vi "toSplitStringArray.vi"(8 "error in (no error)":errorcluster, 9 "editing?":bool=TRUE, 10 "splitIndex":i32, 11 "ScriptEventList in":refnum<class "ScriptEventList.lvclass">) -> (0 "error out":errorcluster, 1 "AfterIndex":string[][](array[string]), 2 "BeforeIndex":string[][](array[string]), 3 "ScriptEventList out":refnum<class "ScriptEventList.lvclass">, 4 "indexedScriptEvent":refnum<class "ScriptEvent.lvclass">)   [LabVIEW 2009, in "Tools.lvlib" / "Scripting.lvlib" / "ScriptEventList.lvclass"]
uses:
  ScriptEventList.lvclass
  ScriptEvent.lvclass
  ScriptEventList.lvclass/ScriptEventList.ctl
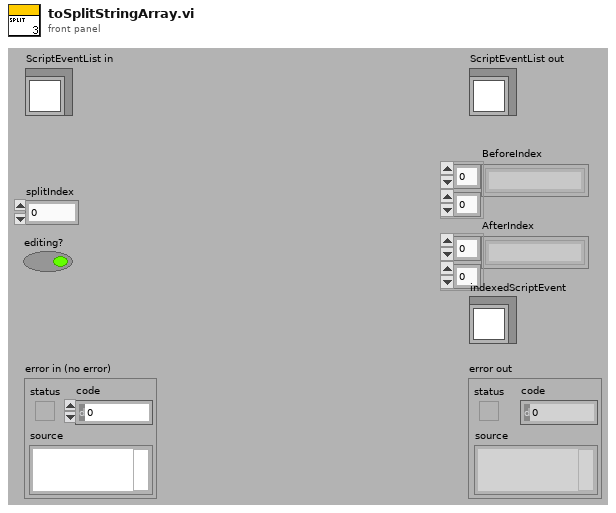
[diagram p1: front panel]
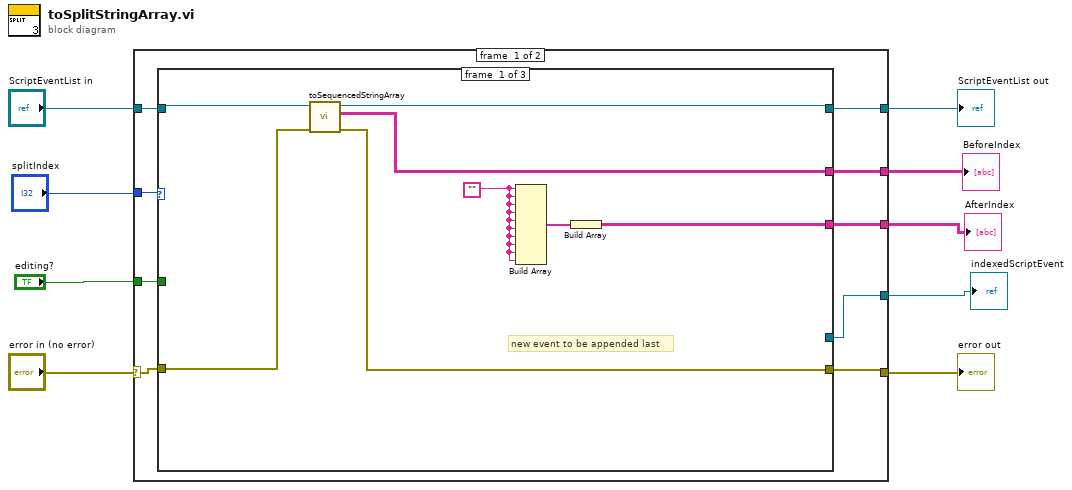
[diagram p0: block diagram]
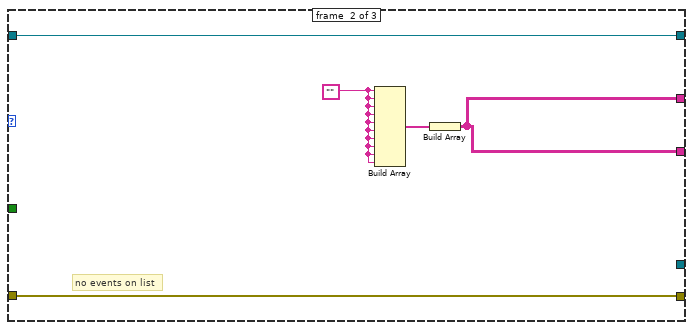
[diagram p2: hidden frame]
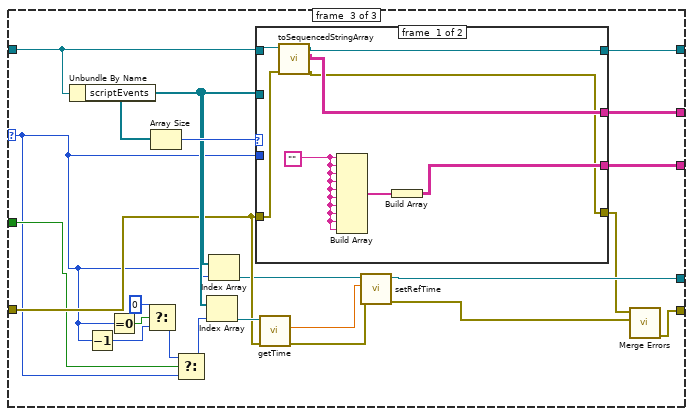
[diagram p3: hidden frame]
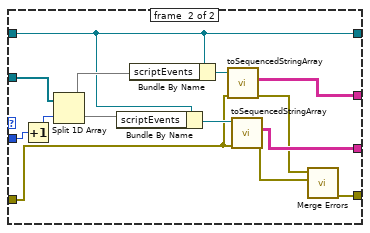
[diagram p4: hidden frame]
diagram:
  n1 = case shown="No Error" "error in (no error)" {
    selector: "error in (no error)" -> [w15 w77]
    tunnel: [w14 w77] -> w8
    tunnel: [w16 w76] -> w6
    tunnel: "ScriptEventList in" -> [w17 w76]
    tunnel: "splitIndex" -> [w18 _]
    tunnel: [w13 _] -> w5
    tunnel: [w12 _] -> w4
    tunnel: [w11 _] -> w3
    tunnel: "editing?" -> [w10 _]
    frame #0 {
      n2 = case shown="0, Default" w18 {
        selector: w18 -> [_ _ w32]
        tunnel: w17 -> [w23 w30 w52]
        tunnel: [w21 w30 w50] -> w16
        tunnel: w15 -> [w22 w31 w46]
        tunnel: [w19 w31 w39] -> w14
        tunnel: [w20 w27 w51] -> w13
        tunnel: [w24 w27 w53] -> w12
        tunnel: [_ _ w42] -> w11
        tunnel: w10 -> [_ _ w38]
        frame #0 {
          w26 = ""
          # "new event to be appended last"
          n3 = call "toSequencedStringArray.vi"("error in (no error)"=w22, "ScriptEventList in"=w23) -> ("error out"=w19:errorcluster, "Array"=w20:string[][], "ScriptEventList out"=w21:refnum<class "ScriptEventList.lvclass">)  [unwired: 7 in]
          n4 = Build Array(w26, w26, w26, w26, w26, w26, w26, w26, w26, w26) -> (w25:string[])
          n5 = Build Array(w25) -> (w24:string[][])
        }
        frame #1 {
          w29 = ""
          # "no events on list"
          n6 = Build Array(w29, w29, w29, w29, w29, w29, w29, w29, w29, w29) -> (w28:string[])
          n7 = Build Array(w28) -> (w27:string[][])
        }
        frame #2 {
          n8 = Unbundle By Name(w52) -> ("scriptEvents"=w48:refnum<class "ScriptEvent.lvclass">[])
          n9 = Decrement(x=w32) -> (x-1=w35:i32)
          n10 = Equal To 0?(x=w32) -> (x = 0?=w33:bool)
          n11 = Select(t=0, s=w33, f=w35) -> (s? t:f=w34:i32)
          n12 = Array Size(array=w48) -> (size(s)=w49:i32)
          n13 = Select(t=w34, s=w38, f=w32) -> (s? t:f=w37:i32)
          n14 = Index Array(array=w48, index=w37) -> (element=w47:refnum<class "ScriptEvent.lvclass">)
          n15 = Index Array(array=w48, index=w32) -> (element=w45:refnum<class "ScriptEvent.lvclass">)
          n16 = case shown="2, Default" w49 {
            tunnel: [w59 w67] -> w53
            tunnel: w52 -> [w58 w70]
            tunnel: w46 -> [w55 w68]
            tunnel: [w56 w71] -> w51
            tunnel: [w57 w70] -> w50
            tunnel: w48 -> [_ w75]
            tunnel: [w54 w64] -> w40
            tunnel: w32 -> [_ w63]
            frame #0 {
              w61 = ""
              n17 = call "toSequencedStringArray.vi"("error in (no error)"=w55, "ScriptEventList in"=w58) -> ("error out"=w54:errorcluster, "Array"=w56:string[][], "ScriptEventList out"=w57:refnum<class "ScriptEventList.lvclass">)  [unwired: 7 in]
              n18 = Build Array(w61, w61, w61, w61, w61, w61, w61, w61, w61, w61) -> (w60:string[])
              n19 = Build Array(w60) -> (w59:string[][])
            }
            frame #1 {
              n20 = Increment(x=w63) -> (x+1=w62:i32)
              n21 = Split 1D Array(array=w75, index=w62) -> (first subarray=w74:refnum<class "ScriptEvent.lvclass">[], second subarray=w72:refnum<class "ScriptEvent.lvclass">[])
              n22 = Bundle By Name(cluster=w70, "scriptEvents"=w72) -> (w69:refnum<class "ScriptEventList.lvclass">)
              n23 = Bundle By Name(cluster=w70, "scriptEvents"=w74) -> (w73:refnum<class "ScriptEventList.lvclass">)
              n24 = call "toSequencedStringArray.vi"("error in (no error)"=w68, "ScriptEventList in"=w73) -> ("error out"=w66:errorcluster, "Array"=w71:string[][])  [unwired: 7 in, 1 out]
              n25 = call "toSequencedStringArray.vi"("error in (no error)"=w68, "ScriptEventList in"=w69) -> ("error out"=w65:errorcluster, "Array"=w67:string[][])  [unwired: 7 in, 1 out]
              n26 = call <vilib>:"Merge Errors.vi"("error in 2 (no error)"=w65, "error in 1 (no error)"=w66) -> ("error out"=w64:errorcluster)  [unwired: 5 in]
            }
          }
          n27 = call "getTime.vi"("error in (no error)"=w46, "ScriptEvent.lvclass in"=w47) -> ("error out"=w43:errorcluster, "time"=w44:dbl)  [unwired: 7 in, 1 out]
          n28 = call "setRefTime.vi"("error in (no error)"=w43, "refTime"=w44, "ScriptEvent.lvclass in"=w45) -> ("error out"=w41:errorcluster, "ScriptEvent.lvclass out"=w42:refnum<class "ScriptEvent.lvclass">)  [unwired: 7 in]
          n29 = call <vilib>:"Merge Errors.vi"("error in 2 (no error)"=w41, "error in 1 (no error)"=w40) -> ("error out"=w39:errorcluster)  [unwired: 5 in]
        }
      }
    }
    frame #1 {
    }
  }
  "error out" <- w8
  "ScriptEventList out" <- w6
  "BeforeIndex" <- w5
  "AfterIndex" <- w4
  "indexedScriptEvent" <- w3
